vi "Example Graph.vi"() -> ()   [LabVIEW 2010]
uses:
  C:/tf/play/labview/Tinkerforge.dll
  Tinkerforge.dll
panel:
  in  "stop":bool
  out "graph":i32[](graph)
  in  "uid":string="amb"
  in  "port":i32=4223
  in  "host":string="localhost"
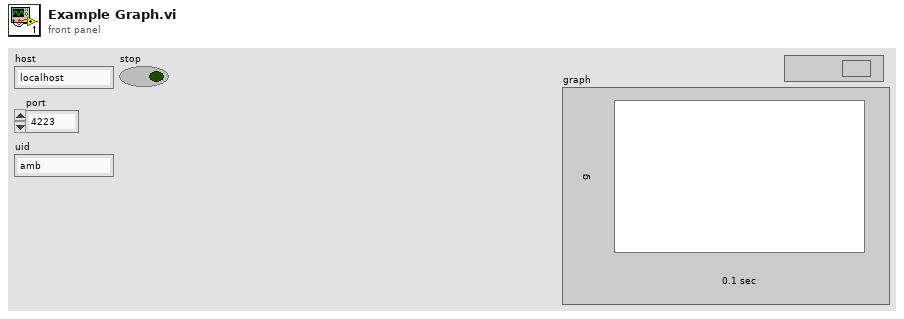
[diagram p1: front panel]
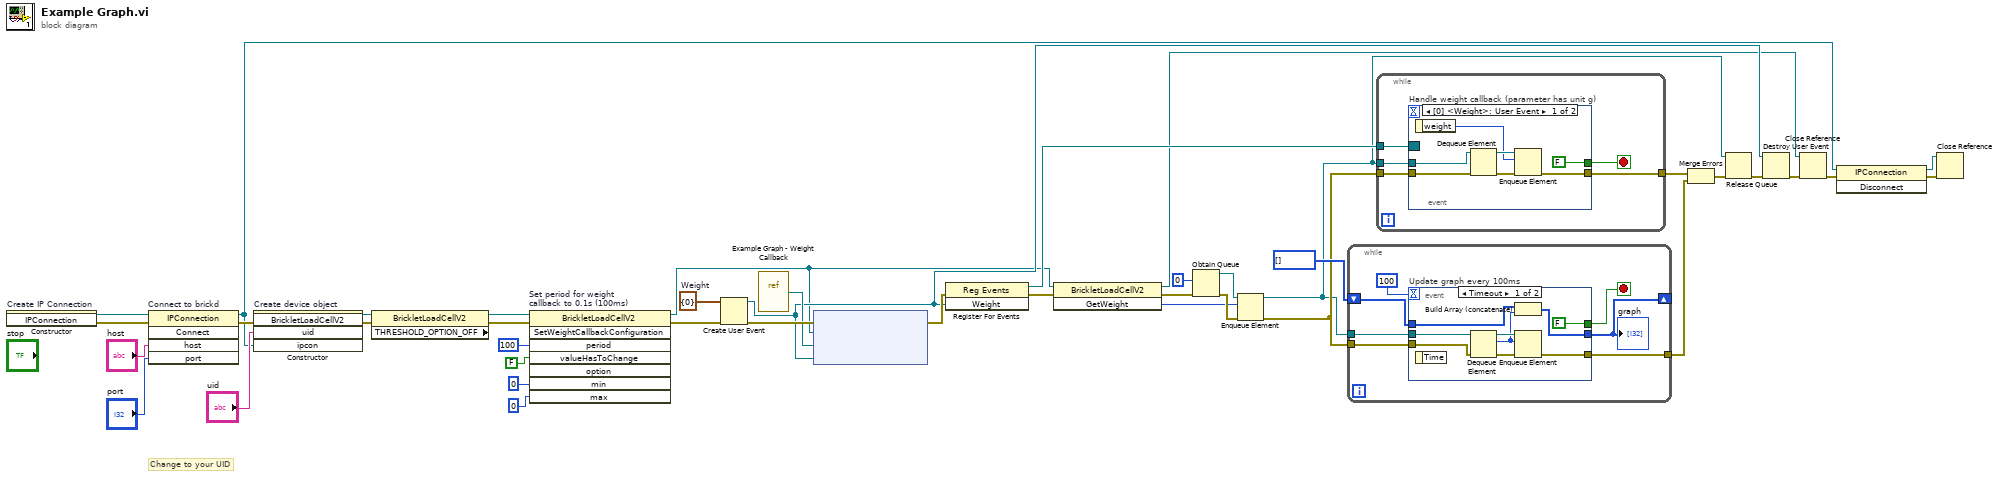
[diagram p0: block diagram]
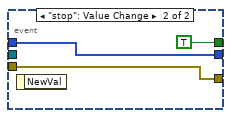
[diagram p2: hidden frame]
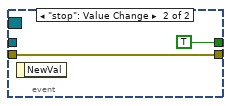
[diagram p3: hidden frame]
diagram:
  w26 = cluster{"weight":i32} {"weight"=0}  # Weight
  # "Change to your UID"
  n1 = constructor on="Create IP Connection" class="IPConnection"() -> (reference out=w41:refnum<k24>, error out=w13:errorcluster)  [unwired: 3 in, 1 out]
  n2 = invoke on="Connect to brickd" class="IPConnection" method="Connect"(reference=w41, error in=w13, "host"="host", "port"="port") -> (reference out=w34:refnum<k24>, error out=w37:errorcluster)  [unwired: 1 in, 3 out]
  n3 = constructor on="Create device object" class="BrickletLoadCellV2"(error in=w37, "uid"="uid", "ipcon"=w34) -> (reference out=w2:refnum<k24>, error out=w3:errorcluster)  [unwired: 2 in, 3 out]
  n4 = property class="BrickletLoadCellV2" props=["THRESHOLD_OPTION_OFF"](reference=w2, error in=w3) -> (reference out=w1:refnum<k24>, error out=w4:errorcluster)  [unwired: 1 out]
  n5 = invoke on="Set period for weight\ncallback to 0.1s (100ms)" class="BrickletLoadCellV2" method="SetWeightCallbackConfiguration"(reference=w1, error in=w4, "period"=i64 100, "valueHasToChange"=FALSE, "min"=0, "max"=0) -> (reference out=w10:refnum<k24>, error out=w25:errorcluster)  [unwired: 2 in, 6 out]
  n6 = Create User Event(user event datatype=w26, error in=w25) -> (user event=w28:refnum<user-event>, error out=w32:errorcluster)
  n7 = vi-ref "Example Graph - Weight Callback.vi"() -> ("vi reference"=w30:refnum<vi>)
  n8 = node ("Register Event Callback")(w32, w10, w30, w28) -> (w31:errorcluster)  [unwired: 1 in, 1 out]
  n9 = register-events(error in=w31, w28) -> (reference out=w29:refnum<event-registration>, error out=w12:errorcluster)  [unwired: 1 in]
  n10 = invoke class="BrickletLoadCellV2" method="GetWeight"(reference=w10, error in=w12) -> (reference out=w9:refnum<k24>, error out=w11:errorcluster, "GetWeight"=w8:i32)  [unwired: 1 in]
  n11 = Obtain Queue(element data type=0, error in (no error)=w11) -> (queue out=w17:refnum<queue>, error out=w19:errorcluster)  [unwired: 3 in, 1 out]
  n12 = Enqueue Element(queue=w17, element=w8, error in (no error)=w19) -> (queue out=w14:refnum<queue>, error out=w18:errorcluster)  [unwired: 1 in, 1 out]
  n13 = while {
    tunnel: [w44] -> w23
    tunnel: w18 -> [w45]
    shift-right: [w46] -> _
    shift-left: i32[] [] -> [w47]
    tunnel: w14 -> [w43]
    stop <- w42 stop-if-true
    n14 = event "Update graph every 100ms" shown="[0] Timeout" {
      selector: _ -> [_ _]
      dyn-events: _ -> [_ _]
      timeout: 100 -> [_ _]
      tunnel: [w57 w59] -> w46
      tunnel: w47 -> [w50 w59]
      tunnel: w45 -> [w56 w58]
      tunnel: [w53 w58] -> w44
      tunnel: w43 -> [w55 _]
      tunnel: [FALSE TRUE] -> w42
      event Timeout {
        n15 = event-data() -> ()  [unwired: 1 in, 1 out]
        n16 = Dequeue Element(queue=w55, error in (no error)=w56) -> (queue out=w52:refnum<queue>, element=w51:i32, error out=w54:errorcluster)  [unwired: 1 in, 1 out]
        n17 = Build Array (concatenate)(w50, w51) -> (w57:i32[])
        n18 = Enqueue Element(queue=w52, element=w51, error in (no error)=w54) -> (error out=w53:errorcluster)  [unwired: 1 in, 2 out]
      }
      event "stop": Value Change {
        n19 = event-data() -> ()  [unwired: 1 in, 1 out]
      }
    }
    "graph" <- w46
  }
  n20 = while {
    tunnel: w29 -> [w65]
    tunnel: [w63] -> w22
    tunnel: w18 -> [w64]
    tunnel: w14 -> [w62]
    stop <- w61 stop-if-true
    n21 = event "Handle weight callback (parameter has unit g)" shown="[0] <Weight>: User Event" {
      selector: w65 -> [_ _]
      dyn-events: _ -> [_ _]
      timeout: _ -> [_ _]
      tunnel: w64 -> [w72 w73]
      tunnel: [w70 w73] -> w63
      tunnel: w62 -> [w69 _]
      tunnel: [FALSE TRUE] -> w61
      event User Event {
        n22 = event-data() -> ("weight"=w66:i32)  [unwired: 1 in]
        n23 = Dequeue Element(queue=w69, error in (no error)=w72) -> (queue out=w68:refnum<queue>, error out=w71:errorcluster)  [unwired: 1 in, 2 out]
        n24 = Enqueue Element(queue=w68, element=w66, error in (no error)=w71) -> (error out=w70:errorcluster)  [unwired: 1 in, 2 out]
      }
      event "stop": Value Change {
        n25 = event-data() -> ()  [unwired: 1 in, 1 out]
      }
    }
  }
  n26 = Merge Errors(w22, w23) -> (w16:errorcluster)
  n27 = Release Queue(queue=w14, error in (no error)=w16) -> (error out=w15:errorcluster)  [unwired: 1 in, 2 out]
  n28 = Destroy User Event(user event=w28, error in=w15) -> (error out=w27:errorcluster)
  n29 = Close Reference(reference=w9, error in (no error)=w27) -> (error out=w36:errorcluster)
  n30 = invoke class="IPConnection" method="Disconnect"(reference=w34, error in=w36) -> (reference out=w33:refnum<k24>, error out=w35:errorcluster)  [unwired: 1 in, 1 out]
  n31 = Close Reference(reference=w33, error in (no error)=w35) -> ()  [unwired: 1 out]
